vi "test write setpoints.vi"() -> ()   [LabVIEW 2015]
uses:
  setpoints.ctl
  backwash.ctl
  coag.ctl
  model type.ctl
  ini.ctl
  file paths.ctl
panel:
  out "Setpoints out":T1={"graph data interval (s)"=100.0, "sludge flow [L/s]"=0.0, "plant flow [L/s]"=0.0, "Plant Flow PID "={"proportional gain (Kc)"=0.05, "integral time (Ti, min)"=1.0, "derivative time (Td, min)"=0.01}, "Sludge PID "={"proportional gain (Kc)"=0.07, "integral time (Ti, min)"=1.0, "derivative time (Td, min)"=0.01}, "backwash"={"Filtered quality target [NTU]"=0.3, "min filtration time [s]"=600.0, "Ripen time [s]"=600.0}, "Coagulant"={"flocculator volume (L)"=0.0, "clarifier volume (L)"=0.0, "dose updates per HRT"=100, "target clarified turbidity (NTU)"=0.3, "Coagulant mode"=enum."manual", "Coag dose [mg/L]"=0.0, "pump mL/rev"=0.0}} {"Coagulant"."target clarified turbidity (NTU)" min=0.1 max=5.0 step=0.01; "Coagulant"."dose updates per HRT" min=1 max=1000 step=1; "Sludge PID"."derivative time (Td, min)" format="%.3f"; "Sludge PID"."integral time (Ti, min)" format="%.3f"; "Sludge PID"."proportional gain (Kc)" format="%.3f"; "Plant Flow PID"."derivative time (Td, min)" format="%.3f"; "Plant Flow PID"."integral time (Ti, min)" format="%.3f"; "Plant Flow PID"."proportional gain (Kc)" format="%.3f"; "plant flow [L/s]" min=0.05 max=1.0 step=0.05; "sludge flow [L/s]" min=0.0 max=0.05 step=0.001; "graph data interval (s)" min=1 max=1000 step=1}
  in  "setpoints":T1={"graph data interval (s)"=100.0, "sludge flow [L/s]"=0.0, "plant flow [L/s]"=0.0, "Plant Flow PID "={"proportional gain (Kc)"=0.05, "integral time (Ti, min)"=1.0, "derivative time (Td, min)"=0.01}, "Sludge PID "={"proportional gain (Kc)"=0.07, "integral time (Ti, min)"=1.0, "derivative time (Td, min)"=0.01}, "backwash"={"Filtered quality target [NTU]"=0.3, "min filtration time [s]"=600.0, "Ripen time [s]"=600.0}, "Coagulant"={"flocculator volume (L)"=0.0, "clarifier volume (L)"=0.0, "dose updates per HRT"=100, "target clarified turbidity (NTU)"=0.3, "Coagulant mode"=enum."manual", "Coag dose [mg/L]"=0.0, "pump mL/rev"=0.0}} {"Coagulant"."target clarified turbidity (NTU)" min=0.1 max=5.0 step=0.01; "Coagulant"."dose updates per HRT" min=1 max=1000 step=1; "Sludge PID"."derivative time (Td, min)" format="%.3f"; "Sludge PID"."integral time (Ti, min)" format="%.3f"; "Sludge PID"."proportional gain (Kc)" format="%.3f"; "Plant Flow PID"."derivative time (Td, min)" format="%.3f"; "Plant Flow PID"."integral time (Ti, min)" format="%.3f"; "Plant Flow PID"."proportional gain (Kc)" format="%.3f"; "plant flow [L/s]" min=0.05 max=1.0 step=0.05; "sludge flow [L/s]" min=0.0 max=0.05 step=0.001; "graph data interval (s)" min=1 max=1000 step=1}
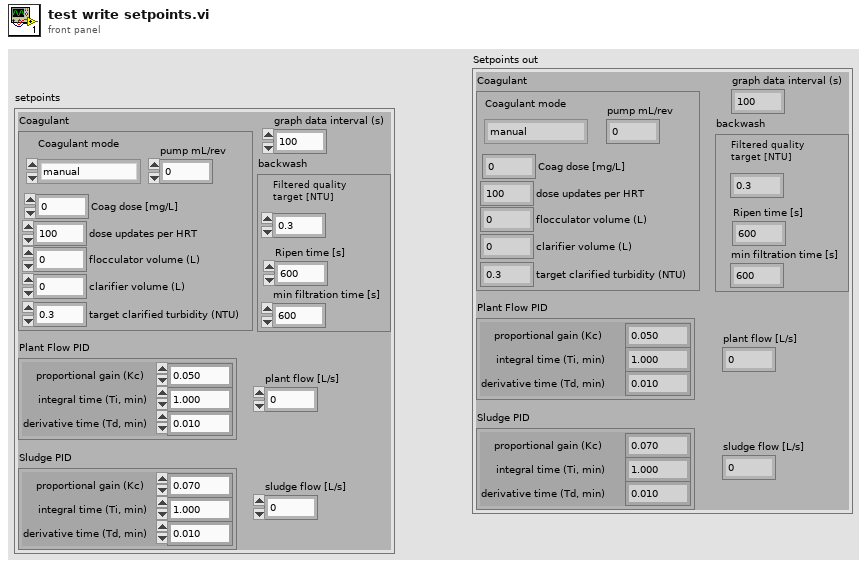
[diagram p1: front panel]
types:
  T1 = typedef "setpoints.ctl" = cluster{"graph data interval (s)":sgl, "sludge flow [L/s]":dbl, "plant flow [L/s]":dbl, "Plant Flow PID ":cluster{"proportional gain (Kc)":dbl, "integral time (Ti, min)":dbl, "derivative time (Td, min)":dbl}, "Sludge PID ":cluster{"proportional gain (Kc)":dbl, "integral time (Ti, min)":dbl, "derivative time (Td, min)":dbl}, "backwash":T2, "Coagulant":T3}
  T2 = typedef "backwash.ctl" = cluster{"Filtered quality target [NTU]":dbl, "min filtration time [s]":dbl, "Ripen time [s]":dbl}
  T3 = typedef "coag.ctl" = cluster{"flocculator volume (L)":dbl, "clarifier volume (L)":dbl, "dose updates per HRT":u32, "target clarified turbidity (NTU)":dbl, "Coagulant mode":T4, "Coag dose [mg/L]":dbl, "pump mL/rev":dbl}
  T4 = typedef "model type.ctl" = enum16{"manual", "simple corrector", "linear regression"}
  T5 = typedef "file paths.ctl" = enum16{"read paths", "close"}
  T6 = typedef "ini.ctl" = enum16{"write", "read"}
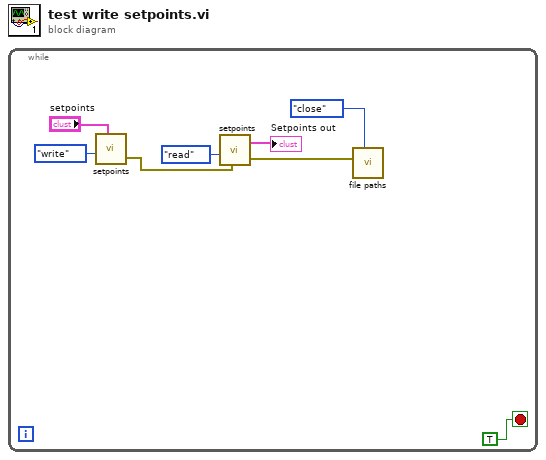
[diagram p0: block diagram]
diagram:
  n1 = while {
    stop <- TRUE stop-if-true
    n2 = call "setpoints.vi"("setpoints"="setpoints", "ini"=ini."write") -> ("error out"=w4:errorcluster)  [unwired: 8 in, 1 out]
    n3 = call "setpoints.vi"("error in (no error)"=w4, "ini"=ini."read") -> ("error out"=w2:errorcluster, "Setpoints out"=→"Setpoints out":T1)  [unwired: 8 in]
    n4 = call "file paths.vi"("error in (no error)"=w2, "file path control"=file_paths."close") -> ()  [unwired: 6 in, 4 out]
  }
